vi "Z900_navX_Util_EncodeProtocol_UnsignedHundredths.vi"(1 "Unsigned Hundredths (0.00)":dbl[](array[numeric])) -> (0 "Little Endian":u8[](array[numeric]))   [LabVIEW 2019]
uses:
  <vilib>/Rock Robotics/WPI/ThirdParty/Sensors/navX/_Util/Z900_navX_Util_BigEndian_to_LittleEndian.vi
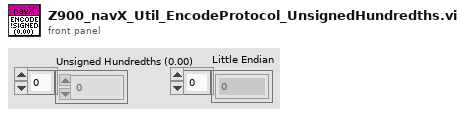
[diagram p1: front panel]
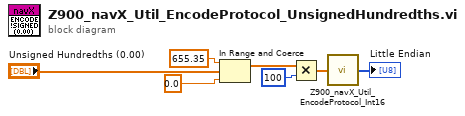
[diagram p0: block diagram]
diagram:
  n1 = In Range and Coerce(upper limit=655.35, x="Unsigned Hundredths (0.00)", lower limit=0.0) -> (coerced(x)=w4:dbl[])  [unwired: 1 out]
  n2 = Multiply(x=w4, y=100) -> (x*y=w6:dbl[])
  n3 = call <vilib>:"Z900_navX_Util_EncodeProtocol_Int16.vi"("Int16"=w6) -> ("Little Endian"=→"Little Endian":u8[])
